vi "Event-Driven State Machine Property Nodes.vi"() -> ()   [LabVIEW 2020]
uses:
  support/States.ctl
  support/State Machine Data.ctl
  <vilib>/DAQmx/read.llb/DAQmx Read (Analog 2D DBL NChan NSamp).vi
  <vilib>/DAQmx/write.llb/DAQmx Write (Analog DBL 1Chan 1Samp).vi
  <vilib>/DAQmx/create/channels.llb/DAQmx Create Channel (AI-Voltage-Basic).vi
  <vilib>/DAQmx/configure/timing.llb/DAQmx Timing (Sample Clock).vi
  <vilib>/DAQmx/miscellaneous.llb/DAQmx Fill In Error Info.vi
  <vilib>/Utility/file.llb/Write Delimited Spreadsheet (DBL).vi
  <vilib>/DAQmx/create/channels.llb/DAQmx Create Channel (AO-Voltage-Basic).vi
panel:
  in  "AO Voltage Channel":tag="PCI-6221/ao1"
  in  "Generate Stimulus":bool
  out "RMS Results Per Channel":dbl[](array[numeric])
  out "Threshold exceeded?":bool
  in  "Acquire":bool
  in  "Samples per channel":i32=100
  in  "Sample Rate (Hz)":dbl=1000.0
  in  "AI Voltage Channel":tag="PCI-6221/ai0, PCI-6221/ai2:3"
  in  "Threshold (rms)":dbl=1.0
  in  "Clear":bool
  in  "Exit":bool
  out "Graph":dbl[][](graph)
  # "Analysis"
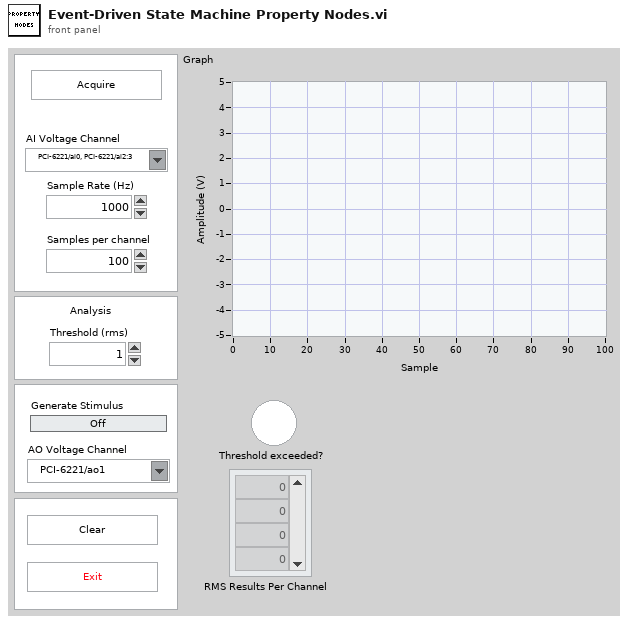
[diagram p1: front panel]
types:
  T1 = typedef "State Machine Data.ctl" = cluster{"Acquisition Data":dbl[][], "Stimulus Value":bool}
  T2 = typedef "States.ctl" = enum16{"Initialize", "Wait for Event", "Acquire", "Analyze", "Log", "Clear", "Update UI", "Update Stumulus", "Exit"}
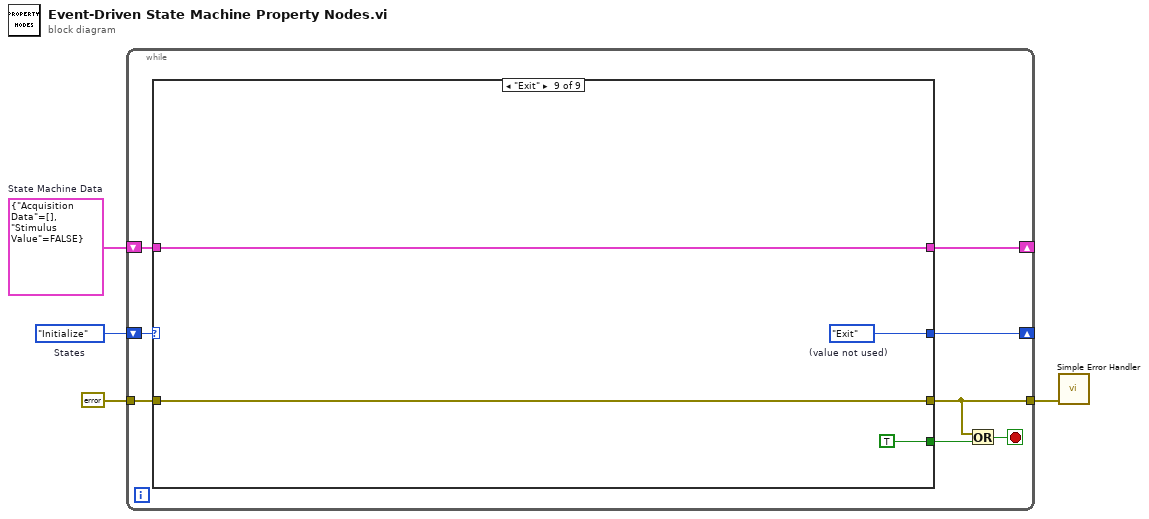
[diagram p0: block diagram]
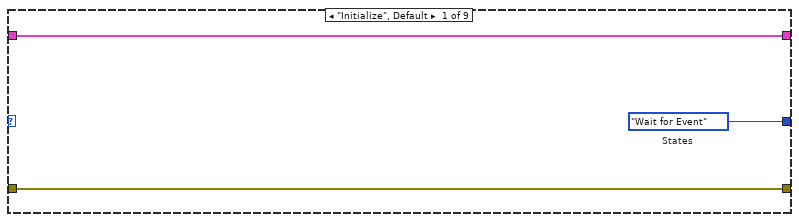
[diagram p2: hidden frame]
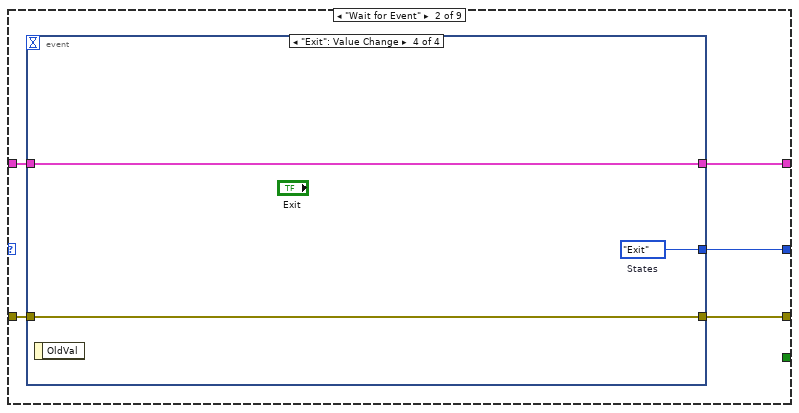
[diagram p3: hidden frame]
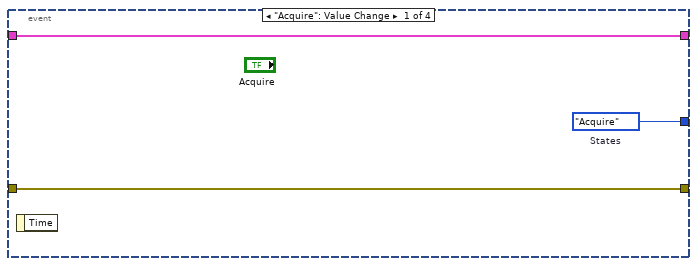
[diagram p4: hidden frame]
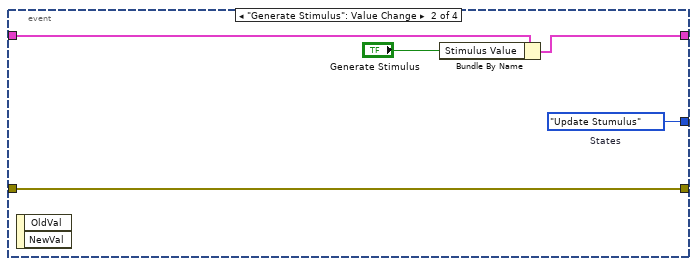
[diagram p5: hidden frame]
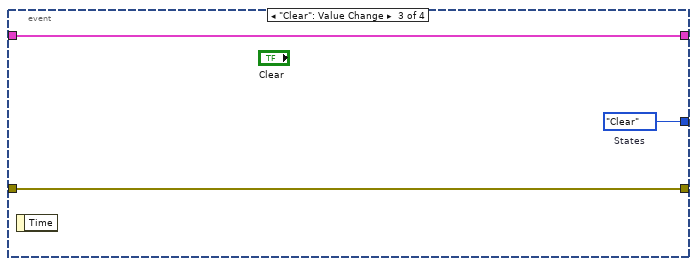
[diagram p6: hidden frame]
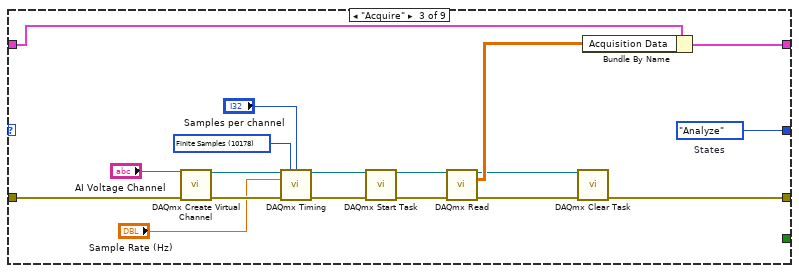
[diagram p7: hidden frame]
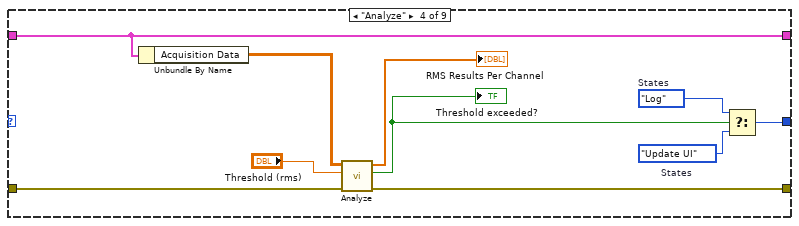
[diagram p8: hidden frame]
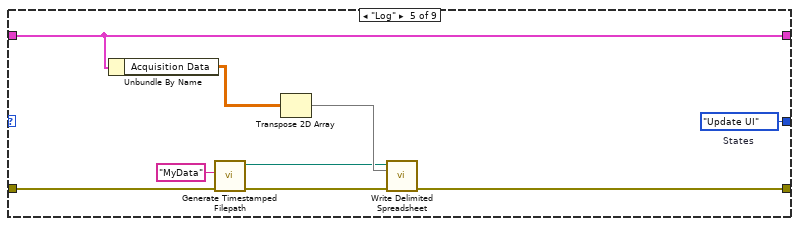
[diagram p9: hidden frame]
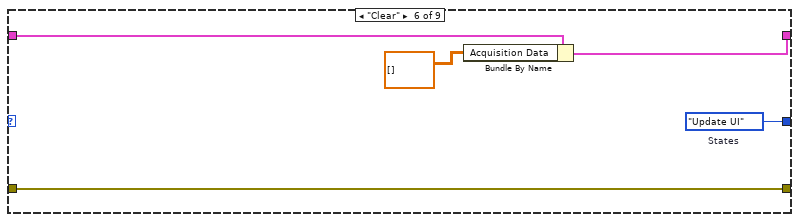
[diagram p10: hidden frame]
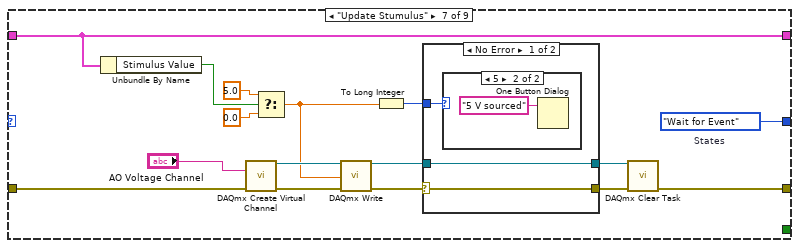
[diagram p11: hidden frame]
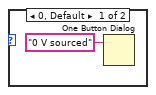
[diagram p12: hidden frame]
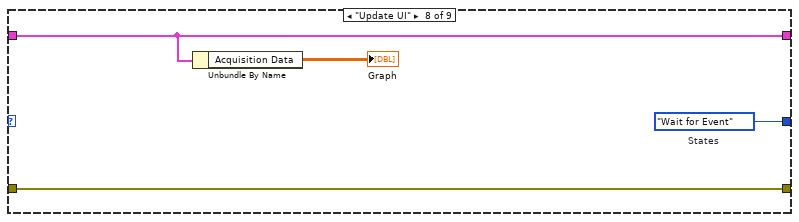
[diagram p14: hidden frame]
diagram:
  w4 = T1 {"Acquisition Data"=[], "Stimulus Value"=FALSE}  # State Machine Data
  w3 = States."Initialize"  # States
  n1 = while {
    tunnel: errorcluster {"status"=FALSE, "code"=0, "source"=""} ("error constant") -> [w11]
    tunnel: [w7] -> w1
    shift-right: [w9] -> _
    shift-left: w4 -> [w10]
    shift-right: [w8] -> _
    shift-left: w3 -> [w12]
    stop <- w6 stop-if-true
    n2 = case shown="\"Exit\"" w12 {
      tunnel: w11 -> [w15 w18 w52 w61 w70 w76 w82 w102 w106]
      tunnel: [w15 w17 w47 w60 w64 w76 w81 w102 w106] -> w7
      tunnel: [w14 w19 w44 w62 w71 w74 w92 w103 w107] -> w9
      tunnel: w10 -> [w14 w20 w45 w62 w71 w75 w92 w103 w107]
      tunnel: [w13 w16 w46 w56 w63 w72 w83 w101 w104] -> w8
      tunnel: [_ _ _ _ _ _ _ _ TRUE] -> w5
      frame "Initialize", Default {
        w13 = States."Wait for Event"  # States
      }
      frame "Wait for Event" {
        n3 = event shown="[3] \"Exit\": Value Change" {
          selector: _ -> [_ _ _ _]
          dyn-events: _ -> [_ _ _ _]
          timeout: _ -> [_ _ _ _]
          tunnel: w20 -> [w23 w28 w31 w33]
          tunnel: [w23 w27 w31 w33] -> w19
          tunnel: w18 -> [w22 w24 w30 w34]
          tunnel: [w22 w24 w30 w34] -> w17
          tunnel: [w21 w25 w29 w32] -> w16
          event "Acquire": Value Change {
            w21 = States."Acquire"  # States
            n4 = event-data() -> ()  [unwired: 1 in, 1 out]
          }
          event "Generate Stimulus": Value Change {
            w25 = States."Update Stumulus"  # States
            n5 = event-data() -> ()  [unwired: 1 in, 2 out]
            n6 = Bundle By Name(cluster=w28, "Stimulus Value"="Generate Stimulus") -> (w27:T1)
          }
          event "Clear": Value Change {
            w29 = States."Clear"  # States
            n7 = event-data() -> ()  [unwired: 1 in, 1 out]
          }
          event "Exit": Value Change {
            w32 = States."Exit"  # States
            n8 = event-data() -> ()  [unwired: 1 in, 1 out]
          }
        }
      }
      frame "Acquire" {
        w43 = 10178 items=["Finite Samples"=10178, "Continuous Samples"=10123, "Hardware Timed Single Point"=12522] ("sample mode")
        w46 = States."Analyze"  # States
        n9 = call-poly <vilib>:"DAQmx Create Virtual Channel.vi"("physical channels"="AI Voltage Channel", "error in"=w52) -> ("task out"=w38:refnum<k21>, "error out"=w51:errorcluster)  [unwired: 12 in]
        n10 = call-poly <vilib>:"DAQmx Timing.vi"("task/channels in"=w38, "sample mode"=w43, "samples per channel"="Samples per channel", "rate"="Sample Rate (Hz)", "error in"=w51) -> ("task out"=w37:refnum<k21>, "error out"=w50:errorcluster)  [unwired: 9 in]
        n11 = call <vilib>:"DAQmx Start Task.vi"("task/channels in"=w37, "error in"=w50) -> ("task out"=w36:refnum<k21>, "error out"=w49:errorcluster)  [unwired: 12 in]
        n12 = call-poly <vilib>:"DAQmx Read.vi"("task/channels in"=w36, "error in"=w49) -> ("task out"=w35:refnum<k21>, "data"=w39:dbl[][], "error out"=w48:errorcluster)  [unwired: 11 in]
        n13 = call <vilib>:"DAQmx Clear Task.vi"("task in"=w35, "error in"=w48) -> ("error out"=w47:errorcluster)  [unwired: 13 in]
        n14 = Bundle By Name(cluster=w45, "Acquisition Data"=w39) -> (w44:T1)
      }
      frame "Analyze" {
        w57 = States."Update UI"  # States
        w58 = States."Log"  # States
        n15 = Unbundle By Name(w62) -> ("Acquisition Data"=w59:dbl[][])
        n16 = call "Analyze.vi"("Error In"=w61, "Treshold (rms)"="Threshold (rms)", "N-Channel Data (2D DBL)"=w59) -> ("Error Out"=w60:errorcluster, "Threshold exceeded?"=w53:bool, "N-Channel Data RMS Results"=→"RMS Results Per Channel":dbl[])  [unwired: 5 in, 1 out]
        "Threshold exceeded?" <- w53
        n17 = Select(t=w58, s=w53, f=w57) -> (s? t:f=w56:T2)
      }
      frame "Log" {
        w63 = States."Update UI"  # States
        n18 = Unbundle By Name(w71) -> ("Acquisition Data"=w68:dbl[][])
        n19 = call "Generate Timestamped Filepath.vi"("Error In"=w70, "appended filename"="MyData") -> ("Error Out"=w65:errorcluster, "timestamped relative filepath"=w66:path)  [unwired: 8 in]
        n20 = Transpose 2D Array(2D array=w68) -> (transposed array=w67:dbl[][])
        n21 = call-poly <vilib>:"Write Delimited Spreadsheet.vi"("file path (dialog if empty)"=w66, "2D data"=w67, "error in (no error)"=w65) -> ("error out"=w64:errorcluster)  [unwired: 11 in, 1 out]
      }
      frame "Clear" {
        w72 = States."Update UI"  # States
        n22 = Bundle By Name(cluster=w75, "Acquisition Data"=dbl[][] []) -> (w74:T1)
      }
      frame "Update Stumulus" {
        w83 = States."Wait for Event"  # States
        n23 = Unbundle By Name(w92) -> ("Stimulus Value"=w84:bool)
        n24 = call-poly <vilib>:"DAQmx Create Virtual Channel.vi"("physical channels"="AO Voltage Channel", "error in"=w82) -> ("task out"=w89:refnum<k21>, "error out"=w88:errorcluster)  [unwired: 12 in]
        n25 = Select(t=5.0, s=w84, f=0.0) -> (s? t:f=w86:dbl)
        n26 = call-poly <vilib>:"DAQmx Write.vi"("task/channels in"=w89, "data"=w86, "error in"=w88) -> ("task out"=w79:refnum<k21>, "error out"=w80:errorcluster)  [unwired: 10 in, 1 out]
        n27 = To Long Integer(number=w86) -> (32bit integer=w85:i32)
        n28 = case shown="No Error" w80 {
          selector: w80 -> [w93 w98]
          tunnel: w85 -> [w95 _]
          tunnel: w79 -> [w94 w99]
          tunnel: [w94 w99] -> w78
          tunnel: [w93 w98] -> w77
          frame No Error {
            n29 = case shown="5" w95 {
              frame 0, Default {
                n30 = One Button Dialog(message="0 V sourced") -> ()  [unwired: 1 in, 1 out]
              }
              frame 5 {
                n31 = One Button Dialog(message="5 V sourced") -> ()  [unwired: 1 in, 1 out]
              }
            }
          }
          frame Error {
          }
        }
        n32 = call <vilib>:"DAQmx Clear Task.vi"("task in"=w78, "error in"=w77) -> ("error out"=w81:errorcluster)  [unwired: 13 in]
      }
      frame "Update UI" {
        w101 = States."Wait for Event"  # States
        n33 = Unbundle By Name(w103) -> ("Acquisition Data"=→"Graph":dbl[][])
      }
      frame "Exit" {
        w104 = States."Exit"  # (value not used)
      }
    }
    n34 = Or(x=w7, y=w5) -> (x .or. y?=w6:bool)
  }
  n35 = call <vilib>:"Simple Error Handler.vi"("error in (no error)"=w1) -> ()  [unwired: 4 in, 5 out]
